vi "Write Pressure Valve.vi"(10 "Pressure Valve":T1, 11 "PressureValve in":refnum<class "PressureValve.lvclass">) -> (3 "PressureValve out":refnum<class "PressureValve.lvclass">)   [LabVIEW 2015]
uses:
  <userlib>/Common/Devices/PressureValve/PressureValve/PressureValve.lvclass
  <userlib>/Common/Devices/PressureValve/Config/PressureValve.ctl
  <userlib>/Common/Devices/PressureValve/PressureValve.lvlib
panel:
  # "dfsfd"
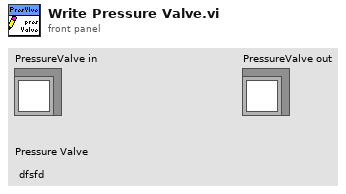
[diagram p1: front panel]
types:
  T1 = typedef "PressureValve.lvlib/PressureValve.ctl" = cluster{}
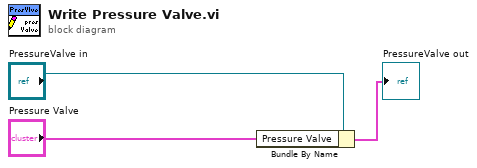
[diagram p0: block diagram]
diagram:
  n1 = Bundle By Name(cluster="PressureValve in", "Pressure Valve"="Pressure Valve") -> (→"PressureValve out":cluster{})
